vi "setChannel.vi"(8 "error in (no error)":errorcluster, 10 "Channel.lvclass":refnum<class "Channel.lvclass">, 11 "RampEvent.lvclass in":refnum<class "RampEvent.lvclass">) -> (0 "error out":errorcluster, 3 "RampEvent.lvclass out":refnum<class "RampEvent.lvclass">)   [LabVIEW 2009, in "Tools.lvlib" / "Scripting.lvlib" / "RampEvent.lvclass"]
uses:
  RampEvent.lvclass
  DatabaseHelpers/Database Objects/Channel/Channel.lvclass
  ScriptEvent.lvclass
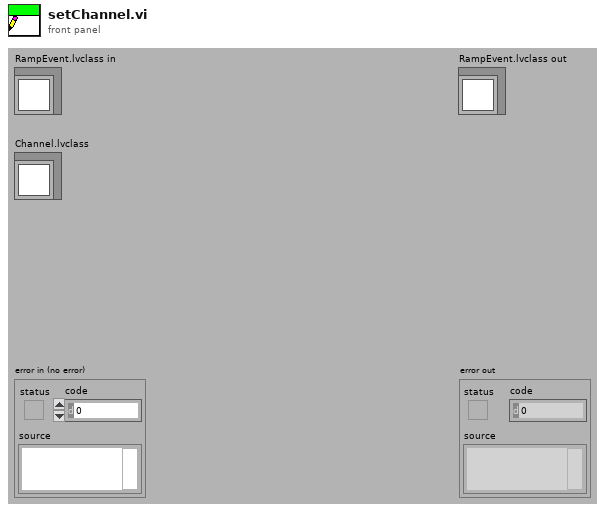
[diagram p1: front panel]
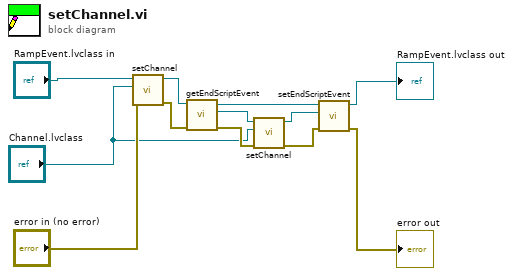
[diagram p0: block diagram]
diagram:
  n1 = call-parent "setChannel.vi"("error in (no error)"="error in (no error)", "Channel.lvclass"="Channel.lvclass", "ScriptEvent.lvclass in"="RampEvent.lvclass in") -> ("error out"=w2:errorcluster, "ScriptEvent.lvclass out"=w10:refnum<class "RampEvent.lvclass">)  [unwired: 7 in]
  n2 = call "getEndScriptEvent.vi"("error in (no error)"=w2, "RampEvent.lvclass in"=w10) -> ("error out"=w4:errorcluster, "ScriptEvent.lvclass"=w7:refnum<class "ScriptEvent.lvclass">, "RampEvent.lvclass out"=w9:refnum<class "RampEvent.lvclass">)  [unwired: 7 in]
  n3 = call-parent "setChannel.vi"("error in (no error)"=w4, "Channel.lvclass"="Channel.lvclass", "ScriptEvent.lvclass in"=w7) -> ("error out"=w5:errorcluster, "ScriptEvent.lvclass out"=w6:refnum<class "ScriptEvent.lvclass">)  [unwired: 7 in]
  n4 = call "setEndScriptEvent.vi"("error in (no error)"=w5, "endScriptEvent.lvclass"=w6, "RampEvent.lvclass in"=w9) -> ("error out"=→"error out":errorcluster, "RampEvent.lvclass out"=→"RampEvent.lvclass out":refnum<class "RampEvent.lvclass">)  [unwired: 7 in]
